vi "File_FromXML.vi"(8 "error in (no error)":errorcluster, 11 "XML String":string) -> (0 "error out":errorcluster, 3 "File out":refnum<class "File.lvclass">)   [LabVIEW 2023, in "File.lvclass"]
doc: "Imports from XML a definition of the file class and creates an object accordingly."
uses:
  File.lvclass
  FileAsCluster.ctl
  Group/GroupAsCluster.ctl
  Channel/ChannelAsCluster.ctl
  <vilib>/NI VeriStand/Custom Device API/Data Reference.ctl
  Meta Data.ctl
  <vilib>/NI VeriStand/Custom Device API/Custom Device API.lvlib
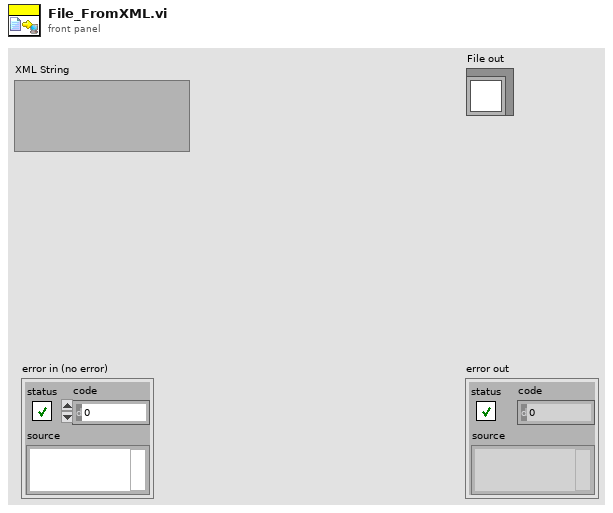
[diagram p1: front panel]
types:
  T1 = typedef "FileAsCluster.ctl" = cluster{"Name":string, "Directory":string, "Date Captured":string, "Groups":T2[], "Meta Data":T5[], "File Start Time":timestamp, "appended path":path}
  T2 = typedef "GroupAsCluster.ctl" = cluster{"Name":string, "Channels":T3[], "Meta Data":T5[]}
  T3 = typedef "ChannelAsCluster.ctl" = cluster{"Name":string, "Data Reference":T4, "Wfm?":bool, "Decimation":i32, "Current Value":dbl, "Meta Data":T5[], "WfmPath":string}
  T4 = typedef "Custom Device API.lvlib/Data Reference.ctl" = i32
  T5 = typedef "Meta Data.ctl" = cluster{"Key":string, "Value":string}
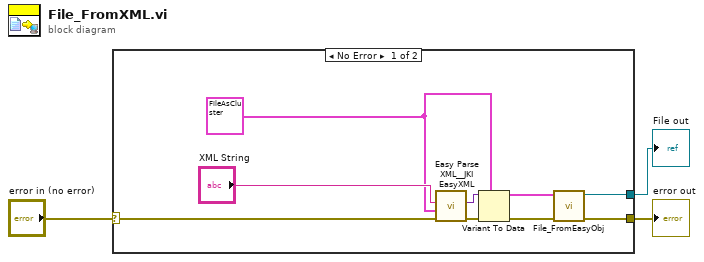
[diagram p0: block diagram]
diagram:
  n1 = case shown="No Error" "error in (no error)" {
    selector: "error in (no error)" -> [w9 w13]
    tunnel: [w5 w13] -> w2
    tunnel: [w6 _] -> w1
    frame No Error {
      w8 = T1 {"Name"="", "Directory"="", "Date Captured"="", "Groups"=[], "Meta Data"=[], "File Start Time"=timestamp(0 s since 1904-01-01), "appended path"=path ""} ("output cluster")
      n2 = call <vilib>:"Easy Parse XML__JKI EasyXML.vi"("error in (no error)"=w9, "LabVIEW Data (Type)"=w8, "XML String"="XML String") -> ("error out"=w10:errorcluster, "LabVIEW Data"=w11:variant)  [unwired: 7 in]
      n3 = Variant To Data(error in=w10, type=w8, Variant=w11) -> (data=w7:T1, error out=w4:errorcluster)
      n4 = call "File_FromEasyObj.vi"("error in (no error)"=w4, "output cluster"=w7) -> ("error out"=w5:errorcluster, "File out"=w6:refnum<class "File.lvclass">)  [unwired: 8 in]
    }
    frame Error {
    }
  }
  "error out" <- w2
  "File out" <- w1
